vi "Self Attributes.vi"(11 "Sender in":refnum<class "Sender.lvclass">) -> (2 "Self Attributes":T1)   [LabVIEW 2020, in "jettl.lvlib" / "Sender.lvlib" / "Sender.lvclass"]
uses:
  Sender.lvclass
  Actor/Attributes.ctl
  Msg/Msg.lvclass
  Actor/Msgs.ctl
  Actor/Actor.lvlib
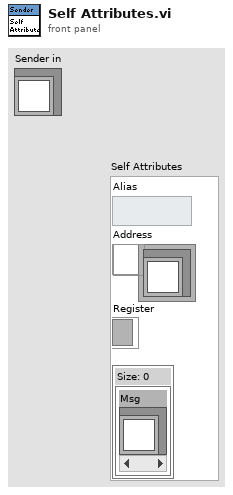
[diagram p1: front panel]
types:
  T1 = typedef "jettl.lvlib/Actor.lvlib/Attributes.ctl" = cluster{"Alias":string, "Address":refnum<user-event>, "Register":refnum<event-registration>, "Implemented Msgs":T2}
  T2 = typedef "jettl.lvlib/Actor.lvlib/Msgs.ctl" = set{refnum<class "Msg.lvclass">}
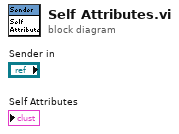
[diagram p0: block diagram]
diagram:
